vi "Controller Main.vi"() -> ()   [LabVIEW 2011]
uses:
  <vilib>/Platform/TimedLoop/XDataNode/timing_clust.ctl
  <vilib>/Platform/TimedLoop/XDataNode/nitl_modes.ctl
  <vilib>/Platform/TimedLoop/XDataNode/wakeup.ctl
  <vilib>/real-time/rtutility.llb/RT Unlock Target (IP).vi
  <vilib>/real-time/rtutility.llb/RT Lock Target (IP).vi
  Controller Global Variables/Controller Status Table.vi
  Controller Global Variables/LNLS Control FOFB Configuration Out.vi
  <vilib>/rtutility.llb/RT Debug String.vi
  <vilib>/Platform/TimedLoop/XDataNode/XDataNode.xnode
  Controller VIs.lvlib
  <vilib>/Platform/TimedLoop/XDataNode/XDNodeRunTimeDep.lvlib
  <vilib>/real-time/NI_Real-Time Libraries.lvlib
  Log VIs.lvlib
  Controller Global Variables.lvlib
panel:
  in  "stop":bool
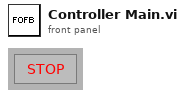
[diagram p1: front panel]
types:
  T1 = cluster{"Operation Mode":enum16{"Idle Mode", "Error Mode", "Manual Mode", "FOFB Mode", "RMM Mode"}, "Correction Period (usec)":i32, "Beam Energy (MeV)":sgl, "Beam Current (mA)":sgl}
  T2 = enum16{"Idle Mode", "Error Mode", "Manual Mode", "FOFB Mode", "RMM Mode"}
  T3 = enum16{"open", "replace", "create", "open or create", "replace or create", "replace or create with confirmation"}
  T4 = typedef "XDNodeRunTimeDep.lvlib/timing_clust.ctl" = cluster{"Expected End [f-1]":u64, "Actual End [f-1]":u64, "Finished Late? [f-1]":bool, "Expected End [i-1]":u64, "Actual End [i-1]":u64, "Finished Late? [i-1]":bool, "Expected Start [i]":u64, "Actual Start [i]":u64, "Expected Start [f]":u64, "Actual Start [f]":u64, "Source Name":string, "Structure Name":string, "Period":i64, "Deadline":i64, "Offset":i64, "Start":i64, "Priority":i32, "Timeout":i32, "Mode":T5, "Wakeup Reason":T6, "Error":errorcluster, "Source Type":string, "Secondary Source Type":string, "Global End Time":u64, "Global Start Time":u64, "Frame Duration":u64, "Iteration Duration":u64, "Assigned CPU":i32, "I/O Scan Engine Mode":u32}
  T5 = typedef "XDNodeRunTimeDep.lvlib/nitl_modes.ctl" = enum32{"No Change", "Process missed periods, maintain original phase", "Discard missed periods, maintain original phase", "Process missed periods, ignore original phase", "Discard missed periods, ignore original phase"}
  T6 = typedef "XDNodeRunTimeDep.lvlib/wakeup.ctl" = enum32{"Normal", "Aborted", "Asynchronous wakeup", "Timing source error", "Timed loop error", "Timeout"}
  T7 = typedef "Type Definitions.lvlib/Type FOFB Configuration.ctl" = cluster{"FOFB Parameters":T8, "Number of Acquisition Chassis":i32, "Number of Actuation Chassis":i32, "Number of BPM Readings":i32, "BPM Reading Names":string[], "Selected BPM Readings":u32[], "Number of Correctors":i32, "Corrector Names":string[], "Selected Correctors":u32[], "Reference Orbit":dbl[], "Response Matrix":dbl[][], "Correction Matrix":dbl[][], "Acquisition Chassis Names":string[], "Actuation Chassis Names":string[], "Acquisition Variables":cluster{"Variable Name":string, "Chassis Name":string}[], "Actuation Variables":cluster{"Variable Name":string, "Chassis Name":string}[], "PS Matrix Mapping":cluster{u32[]}[], "Inverse PS Matrix Mapping":u32[][], "Response Matrix Beam Energy (MeV)":dbl, "PID Parameters":T15[], "BPM Planes":enum8{"H", "V"}[], "Corrector Planes":enum8{"H", "V"}[], "RMM Step Factor":dbl[]}
  T8 = typedef "Type Definitions.lvlib/Type FOFB Parameters.ctl" = cluster{"Network":T9, "Fast Acquisition":T10, "Response Matrix Measurement":T11, "Correction Algorithm":T12, "Acquisition Network":T13, "Actuation Network":T14}
  T9 = typedef "Type Definitions.lvlib/Type Network Configuration.ctl" = cluster{"FOFB Controller IP":string, "LNLS Control Network IP":string, "LNLS Control Network Power Supplies TCP Port":u16, "LNLS Control Network FOFB Configuration TCP Port":u16, "Data Server TCP Port":u16, "Monitoring Data TCP Port":u16, "Configuration GUI TCP Port":u16, "TCP Listening Timeout":i32}
  T10 = typedef "Type Definitions.lvlib/Type FA Configuration.ctl" = cluster{"Acquisition Period":u32, "Data Buffer Size":u32, "Monitoring Period":u32}
  T11 = typedef "Type Definitions.lvlib/Type Response Matrix Measurement Configuration.ctl" = cluster{"Step Amplitude":dbl, "Time Between Steps":u32, "Step Duration":u32, "Number of Averages":u32}
  T12 = typedef "Type Definitions.lvlib/Type Correction Algorithm Configuration.ctl" = cluster{"Correction Period":u32, "Reference Orbit Path":path, "Response Matrix Path":path, "Correction Matrix Path":path, "Horizontal Correction Factor":dbl, "Vertical Correction Factor":dbl, "Beam Current FOFB Threshold":dbl, "Decouple H-V":bool, "Use Additional BPM LPF":bool, "BPM LPF Cutoff":dbl}
  T13 = typedef "Type Definitions.lvlib/Type Acquisition Network Configuration.ctl" = cluster{"Chassis Name":string, "Variables":cluster{"Variable Name":string, "Matrix Order":u32, "Location":dbl, "Plane":enum8{"H", "V"}, "On Correction":bool}[]}[]
  T14 = typedef "Type Definitions.lvlib/Type Actuation Network Configuration.ctl" = cluster{"Chassis Name":string, "Variables":cluster{"Variable Name":string, "Matrix Order":u32, "RMM Step Factor":dbl, "Plane":enum8{"H", "V"}, "On Correction":bool, "Kc":dbl, "Ti":dbl, "Td":dbl}[]}[]
  T15 = typedef "Type Definitions.lvlib/Type PID Parameters.ctl" = cluster{"Kc":fxp<+/-,16,8>, "Ti":fxp<+/-,16,8>, "Td":fxp<+/-,16,8>}
  T16 = typedef "Type Definitions.lvlib/Type PS Variables.ctl" = cluster{"PS Setpoint Variables":refnum<k21>[], "PS Reading Variables":refnum<k21>[], "PS Status Variables":refnum<k21>[], "PS ON-OFF Variables":refnum<k21>[], "PS Enable Variables":refnum<k21>[]}
  T17 = typedef "Type Definitions.lvlib/Type BPM Variables.ctl" = cluster{"BPM Variables":refnum<k21>[]}
  T18 = typedef "Type Definitions.lvlib/Type Synchronization Objects.ctl" = cluster{"Blocking":T19, "Non-blocking":T21}
  T19 = typedef "Type Definitions.lvlib/Type Blocking Synchronization Objects.ctl" = cluster{"FA Request Queue":refnum<queue>, "FA Start Notifier":refnum<notifier>, "FA Finished Queue":refnum<queue>, "FA Finished Broadcast Notifier":refnum<notifier>, "RMM Start FIFO":refnum<k33>, "Monitoring Data Notifier":refnum<notifier>, "Operation Mode Change Request FIFO":refnum<k33>, "Monitoring BPM and PS Data FIFO":refnum<k33>, "FA BPM and PS Data FIFO":refnum<k33>, "PS Manual Setpoints FIFO":refnum<k33>, "PS RMM Setpoints FIFO":refnum<k33>, "Controller Errors FIFO":refnum<k33>, "FA Running Semaphore":T20, "RT Trace Request Queue":refnum<queue>}
  T20 = typedef "Semaphore RefNum" = refnum<k1>
  T21 = typedef "Type Definitions.lvlib/Type Non-blocking Synchronization Objects.ctl" = cluster{"Stop Controller Notifier":refnum<notifier>, "Stop Controller (Time-Critical Loop) FIFO":refnum<k33>, "FA Stop Queue":refnum<queue>, "RMM Finished FIFO":refnum<k33>, "RMM Stop FIFO":refnum<k33>, "FOFB Variables Queue":refnum<queue>, "Diagnostics Data Notifier":refnum<notifier>, "Diagnostics Data (Time-Critical Loop) FIFO":refnum<k33>, "Actuation State Change Request FIFO":refnum<k33>, "FA Diagnostics FIFO":refnum<k33>}
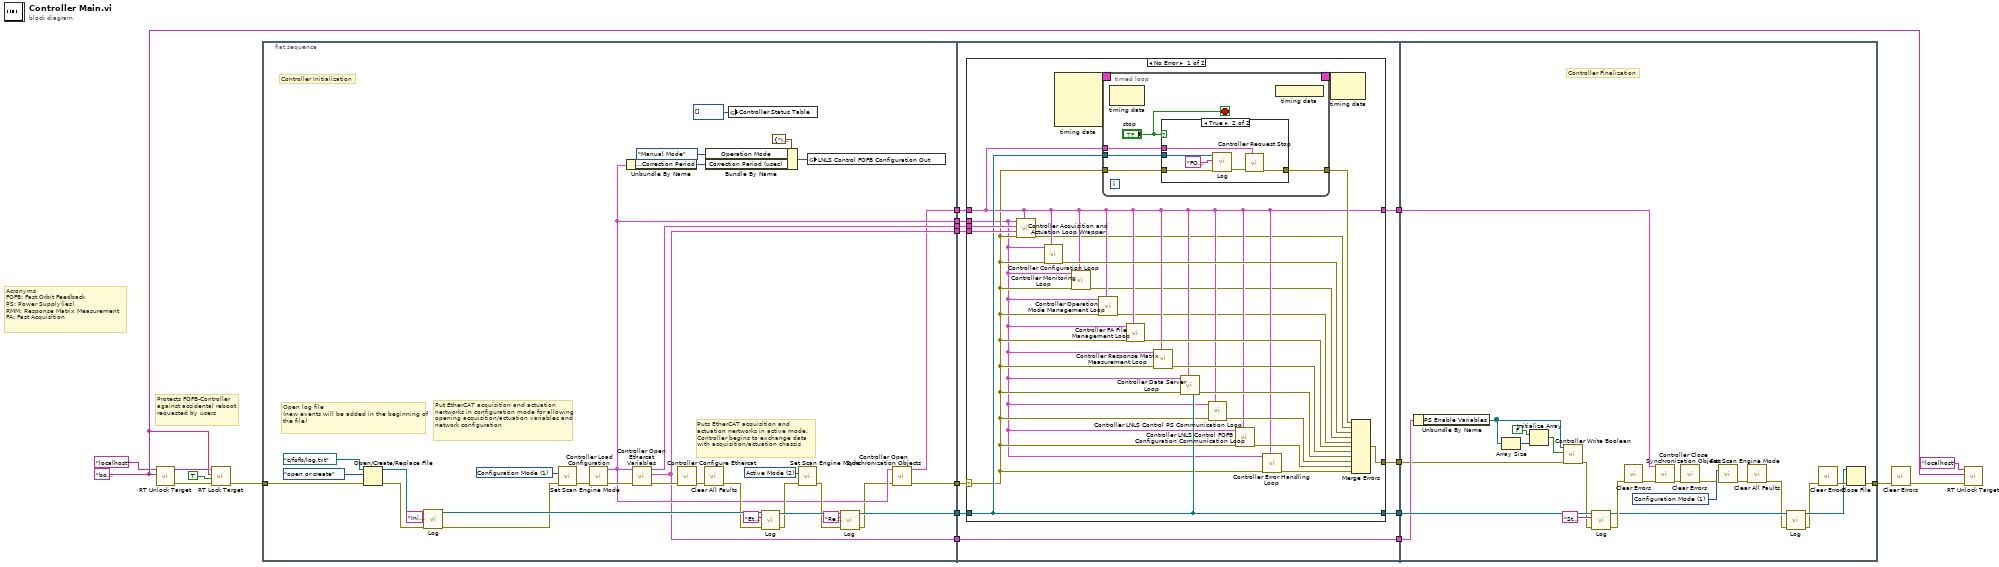
[diagram p0: block diagram]
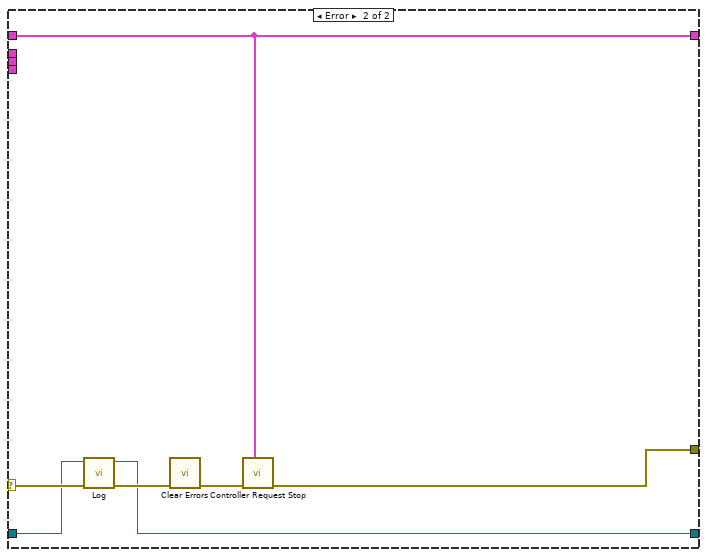
[diagram p3: hidden frame]
diagram:
  w9 = "boo500mev" ("password")
  # "Protects FOFB-Controller against accidental reboot requested by users"
  # "Acronyms\nFOFB: Fast Orbit Feedback\nPS: Power Supply(ies)\nRMM: Response Matrix Measurement\nFA: Fast Acquisition"
  n1 = call-poly <vilib>:"RT Unlock Target.vi"("password"=w9, "target address"="localhost") -> ("error out"=w7:errorcluster, "target address out"=w6:string)  [unwired: 7 in, 1 out]
  n2 = call-poly <vilib>:"RT Lock Target.vi"("error in (no error)"=w7, "password-protect restarts? (F)"=TRUE, "password"=w9, "target address"=w6) -> ("error out"=w3:errorcluster)  [unwired: 6 in, 1 out]
  n3 = flat-sequence {
    tunnel: [w23] -> w20
    tunnel: [w52] -> w19
    tunnel: [w29] -> w18
    tunnel: [w30] -> w17
    tunnel: [w24] -> w16
    tunnel: [w50] -> w15
    tunnel: w3 -> [w51]
    tunnel: [w29] -> w14
    tunnel: w20 -> [w53]
    tunnel: w19 -> [w62]
    tunnel: w18 -> [w61]
    tunnel: w17 -> [w60]
    tunnel: w16 -> [w59]
    tunnel: [w58] -> w13
    tunnel: [w57] -> w12
    tunnel: w15 -> [w56]
    tunnel: [w55] -> w11
    tunnel: [w54] -> w10
    tunnel: w14 -> [w54]
    tunnel: w13 -> [w125]
    tunnel: w12 -> [w109]
    tunnel: w11 -> [w127]
    tunnel: [w126] -> w2
    tunnel: w10 -> [w124]
    frame #0 {
      w33 = 2 items=["Configuration Mode"=1, "Active Mode"=2] ("mode (Active Mode)")
      w47 = 1 items=["Configuration Mode"=1, "Active Mode"=2] ("mode (Active Mode)")
      # "Puts EtherCAT acquisition and actuation nertworks in active mode. Controller begins to exchange data with acquisition/actuation chassis"
      # "Open log file\n(new events will be added in the beginning of the file)"
      # "Controller Initialization"
      # "Put EtherCAT acquisition and actuation nertworks in configuration mode for allowing opening acquisition/actuation variables and network configuration"
      n4 = Open/Create/Replace File(file path (use dialog)=path "c:/fofb/log.txt", error in=w51, operation (0:open)=T3."open or create") -> (refnum out=w46:refnum<file>, error out=w34:errorcluster)  [unwired: 3 in, 1 out]
      n5 = call "Log.vi"("error in (no error)"=w34, "String"="Initializing FOFB-Controller...", "Log File Reference"=w46) -> ("error out"=w31:errorcluster, "Log File Reference"=w37:refnum<file>)  [unwired: 7 in]
      n6 = call <vilib>:"Set Scan Engine Mode.vi"("mode (Active Mode)"=w47, "error in (no error)"=w31) -> ("error out"=w44:errorcluster)  [unwired: 13 in]
      n7 = call "Controller Load Configuration.vi"("error in (no error)"=w44) -> ("error out"=w43:errorcluster, "FOFB Configuration"=w30:T7)  [unwired: 9 in]
      n8 = Unbundle By Name(w30) -> ("FOFB Parameters.Correction Algorithm.Correction Period"=w28:u32)
      n9 = call "Controller Open Ethercat Variables.vi"("error in (no error)"=w43, "FOFB Configuration"=w30) -> ("error out"=w38:errorcluster, "PS Variables"=w29:T16, "BPM Variables"=w52:T17)  [unwired: 7 in]
      n10 = call "Controller Configure Ethercat.vi"("error in (no error)"=w38) -> ("error out"=w42:errorcluster)  [unwired: 10 in]
      n11 = call <vilib>:"Clear All Faults.vi"("error in (no error)"=w42) -> ("error out"=w36:errorcluster)  [unwired: 1 in, 9 out]
      n12 = Bundle By Name(cluster=T1 {"Operation Mode"=enum."Idle Mode", "Correction Period (usec)"=0, "Beam Energy (MeV)"=0.0, "Beam Current (mA)"=0.0} ("LNLS Control FOFB Configuration"), "Operation Mode"=T2."Manual Mode" ("Controller_Operation_Mode"), "Correction Period (usec)"=w28) -> (w25:T1)
      n13 = global write "Controller Status Table.vi" "Controller Status Table"(i32[] [] ("Controller Status Table")) -> ()
      n14 = call "Log.vi"("error in (no error)"=w36, "String"="EtherCAT acquisition and actuation networks entering in active mode...", "Log File Reference"=w37) -> ("error out"=w35:errorcluster, "Log File Reference"=w39:refnum<file>)  [unwired: 7 in]
      n15 = call <vilib>:"Set Scan Engine Mode.vi"("mode (Active Mode)"=w33, "error in (no error)"=w35) -> ("error out"=w32:errorcluster)  [unwired: 13 in]
      n16 = global write "LNLS Control FOFB Configuration Out.vi" "LNLS Control FOFB Configuration Out"(w25) -> ()
      n17 = call "Log.vi"("error in (no error)"=w32, "String"="Reading storage ring status (BPMs and power supplies readings)...", "Log File Reference"=w39) -> ("error out"=w21:errorcluster, "Log File Reference"=w50:refnum<file>)  [unwired: 7 in]
      n18 = call "Controller Open Synchronization Objects.vi"("error in (no error)"=w21, "FOFB Configuration"=w30) -> ("error out"=w23:errorcluster, "Sync Objects"=w24:T18)  [unwired: 8 in]
    }
    frame #1 {
      n19 = case shown="No Error" w53 {
        selector: w53 -> [w66 w105]
        tunnel: w62 -> [w82 _]
        tunnel: w61 -> [w71 _]
        tunnel: w60 -> [w65 _]
        tunnel: w59 -> [w68 w101]
        tunnel: [w68 w101] -> w58
        tunnel: [w81 w99] -> w57
        tunnel: w56 -> [w70 w103]
        tunnel: [w70 w102] -> w55
        frame No Error {
          n20 = call "Controller Acquisition and Actuation Loop Wrapper.vi"("Sync Objects"=w68, "error in (no error)"=w66, "PS Variables"=w71, "BPM Variables"=w82, "FOFB Configuration"=w65) -> ("error out"=w67:errorcluster)  [unwired: 6 in]
          n21 = call "Controller Configuration Loop.vi"("Sync Objects"=w68, "error in (no error)"=w66, "FOFB Configuration"=w65) -> ("error out"=w72:errorcluster)  [unwired: 8 in]
          n22 = node-c288() -> (w80:T4)  [unwired: 4 in]
          n23 = call "Controller Monitoring Loop.vi"("Sync Objects"=w68, "error in (no error)"=w66, "FOFB Configuration"=w65) -> ("error out"=w64:errorcluster)  [unwired: 8 in]
          n24 = call "Controller Operation Mode Management Loop.vi"("Sync Objects"=w68, "error in (no error)"=w66, "FOFB Configuration"=w65) -> ("error out"=w63:errorcluster)  [unwired: 8 in]
          n25 = timed-loop {
            tunnel: w66 -> [w84]
            tunnel: [w83] -> w74
            timing: w80 -> [_]
            timing-out: [_] -> w79
            tunnel: w68 -> [w87]
            tunnel: w70 -> [w85]
            stop <- "stop" stop-if-true
            n26 = node-c288() -> ()  [unwired: 1 in, 1 out]
            n27 = case shown="True" "stop" {
              tunnel: w87 -> [_ w94]
              tunnel: w85 -> [_ w92]
              tunnel: w84 -> [w88 w90]
              tunnel: [w88 w89] -> w83
              frame False {
              }
              frame True {
                n28 = call "Log.vi"("error in (no error)"=w90, "String"="FOFB-Controller stop requested by user...", "Log File Reference"=w92) -> ("error out"=w93:errorcluster)  [unwired: 7 in, 1 out]
                n29 = call "Controller Request Stop.vi"("Sync Objects"=w94, "error in (no error)"=w93) -> ("error out"=w89:errorcluster)  [unwired: 9 in]
              }
            }
            n30 = node-c288() -> ()  [unwired: 1 out]
          }
          n31 = call "Controller FA File Management Loop.vi"("Sync Objects"=w68, "error in (no error)"=w66, "FOFB Configuration"=w65) -> ("error out"=w76:errorcluster)  [unwired: 8 in]
          n32 = call "Controller Response Matrix Measurement Loop.vi"("Sync Objects"=w68, "error in (no error)"=w66, "FOFB Configuration"=w65) -> ("error out"=w73:errorcluster)  [unwired: 8 in]
          n33 = call "Controller Data Server Loop.vi"("Log File Reference"=w70, "Sync Objects"=w68, "error in (no error)"=w66, "FOFB Configuration"=w65) -> ("error out"=w75:errorcluster)  [unwired: 7 in]
          n34 = call "Controller LNLS Control PS Communication Loop.vi"("Sync Objects"=w68, "error in (no error)"=w66, "FOFB Configuration"=w65) -> ("error out"=w77:errorcluster)  [unwired: 8 in]
          n35 = call "Controller LNLS Control FOFB Configuration Communication Loop.vi"("Sync Objects"=w68, "error in (no error)"=w66, "FOFB Configuration"=w65) -> ("error out"=w78:errorcluster)  [unwired: 8 in]
          n36 = call "Controller Error Handling Loop.vi"("Sync Objects"=w68, "error in (no error)"=w66, "FOFB Configuration"=w65) -> ("error out"=w69:errorcluster)  [unwired: 8 in]
          n37 = node-c288(w79) -> ()  [unwired: 1 out]
          n38 = Merge Errors(w74, w67, w72, w64, w63, w76, w73, w75, w77, w78, w69) -> (w81:errorcluster)
        }
        frame Error {
          n39 = call "Log.vi"("error in (no error)"=w105, "Log File Reference"=w103) -> ("error out"=w104:errorcluster, "Log File Reference"=w102:refnum<file>)  [unwired: 8 in]
          n40 = call <vilib>:"Clear Errors.vi"("error in (no error)"=w104) -> ("error out"=w100:errorcluster)  [unwired: 6 in]
          n41 = call "Controller Request Stop.vi"("Sync Objects"=w101, "error in (no error)"=w100) -> ("error out"=w99:errorcluster)  [unwired: 9 in]
        }
      }
    }
    frame #2 {
      w123 = 1 items=["Configuration Mode"=1, "Active Mode"=2] ("mode (Active Mode)")
      # "Controller Finalization"
      n42 = Unbundle By Name(w124) -> ("PS Enable Variables"=w110:refnum<k21>[])
      n43 = Array Size(array=w110) -> (size(s)=w114:i32)
      n44 = Initialize Array(FALSE, w114) -> (w113:bool[])
      n45 = call "Controller Write Boolean.vi"("Error In"=w109, "Values"=w113, "Variables"=w110) -> ("Error Out"=w111:errorcluster)  [unwired: 8 in]
      n46 = call "Log.vi"("error in (no error)"=w111, "String"="Stoppping FOFB-Controller...", "Log File Reference"=w127) -> ("error out"=w120:errorcluster, "Log File Reference"=w119:refnum<file>)  [unwired: 7 in]
      n47 = call <vilib>:"Clear Errors.vi"("error in (no error)"=w120) -> ("error out"=w117:errorcluster)  [unwired: 6 in]
      n48 = call "Controller Close Synchronization Objects.vi"("error in (no error)"=w117, "Sync Objects"=w125) -> ("error out"=w108:errorcluster)  [unwired: 9 in]
      n49 = call <vilib>:"Clear Errors.vi"("error in (no error)"=w108) -> ("error out"=w107:errorcluster)  [unwired: 6 in]
      n50 = call <vilib>:"Set Scan Engine Mode.vi"("mode (Active Mode)"=w123, "error in (no error)"=w107) -> ("error out"=w122:errorcluster)  [unwired: 13 in]
      n51 = call <vilib>:"Clear All Faults.vi"("error in (no error)"=w122) -> ("error out"=w118:errorcluster)  [unwired: 1 in, 9 out]
      n52 = call "Log.vi"("error in (no error)"=w118, "Log File Reference"=w119) -> ("error out"=w106:errorcluster, "Log File Reference"=w116:refnum<file>)  [unwired: 8 in]
      n53 = call <vilib>:"Clear Errors.vi"("error in (no error)"=w106) -> ("error out"=w121:errorcluster)  [unwired: 6 in]
      n54 = Close File(refnum=w116, error in=w121) -> (error out=w126:errorcluster)  [unwired: 1 out]
    }
  }
  n55 = call <vilib>:"Clear Errors.vi"("error in (no error)"=w2) -> ("error out"=w1:errorcluster)  [unwired: 6 in]
  n56 = call-poly <vilib>:"RT Unlock Target.vi"("error in (no error)"=w1, "password"=w9, "target address"="localhost") -> ()  [unwired: 6 in, 3 out]
